vi "etlOpenDynReg.vi"   [LabVIEW 2017]
uses:
  <vilib>/DAQmx/create/channels.llb/DAQmx Create Channel (AO-Voltage-Basic).vi
  globalDevices.vi
  <vilib>/DAQmx/configure/timing.llb/DAQmx Timing (Sample Clock).vi
  <resource>/objmgr/daqmx.rc
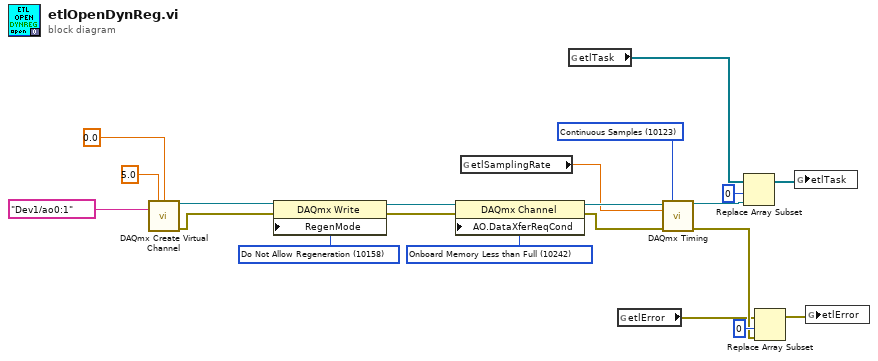
[diagram p0: block diagram]
diagram:
  w10 = 10123 items=["Finite Samples"=10178, "Continuous Samples"=10123, "Hardware Timed Single Point"=12522] ("sample mode")
  w14 = 10242 items=["Onboard Memory Empty"=10235, "Onboard Memory Half Full or Less"=10239, "Onboard Memory Less than Full"=10242] ("AO.DataXferReqCond")
  w17 = 10158 items=["Allow Regeneration"=10097, "Do Not Allow Regeneration"=10158] ("RegenMode")
  n1 = call-poly <vilib>:"DAQmx Create Virtual Channel.vi"("maximum value"=5.0, "minimum value"=0.0, "physical channels"=tag "Dev1/ao0:1") -> ("task out"=w19:refnum<k21>, "error out"=w18:errorcluster)  [unwired: 11 in]
  n2 = property class="DAQmx Write"(reference=w19, error in=w18, "RegenMode"=w17) -> (reference out=w16:refnum<k21>, error out=w15:errorcluster)
  n3 = property class="DAQmx Channel"(reference=w16, error in=w15, "AO.DataXferReqCond"=w14) -> (reference out=w13:refnum<k21>, error out=w12:errorcluster)
  n4 = global read "globalDevices.vi" "etlSamplingRate"() -> (w11:dbl)
  n5 = global read "globalDevices.vi" "etlTask"() -> (w8:refnum<k21>[])
  n6 = global read "globalDevices.vi" "etlError"() -> (w1:errorcluster[])
  n7 = call-poly <vilib>:"DAQmx Timing.vi"("task/channels in"=w13, "sample mode"=w10, "rate"=w11, "error in"=w12) -> ("task out"=w6:refnum<k21>, "error out"=w2:errorcluster)  [unwired: 10 in]
  n8 = Replace Array Subset(array=w8, new element=w6, index=0) -> (w5:refnum<k21>[])
  n9 = Replace Array Subset(array=w1, new element=w2, index=0) -> (w4:errorcluster[])
  n10 = global write "globalDevices.vi" "etlTask"(w5) -> ()
  n11 = global write "globalDevices.vi" "etlError"(w4) -> ()
